vi "Trim Both Whitespace.vi"(0 "String":string) -> (2 "Trimmed String":string)   [LabVIEW 2017, in "Communicable State Machine.lvlib"]
doc: "### Trim Both Whitespace.vi\n\nRemove all ASCII whitespace characters (spaces, tabs, carriage returns, and line feeds) from the beginning, end, or both.\n\n-- <b>Controls</b> --\n- <b>string</b>: String to be processed\n\n-- <b>Indicators</b> --\n- <b>trimmed string</b>: Processed string"
uses:
  Communicable State Machine.lvlib
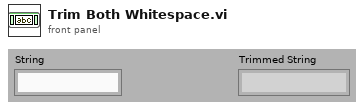
[diagram p1: front panel]
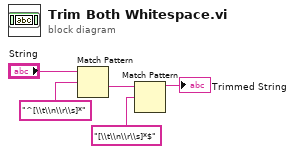
[diagram p0: block diagram]
diagram:
  n1 = Match Pattern(string="String", regular expression="^[\\t\\n\\r\\s]*") -> (after substring=w3:string)  [unwired: 1 in, 3 out]
  n2 = Match Pattern(string=w3, regular expression="[\\t\\n\\r\\s]*$") -> (before substring=→"Trimmed String":string)  [unwired: 1 in, 3 out]
